vi "Test Publisher.vi"() -> ()   [LabVIEW 2021]
uses:
  ChannelCommon/typedef/FIFO Config.ctl
  ChannelCommon/ChannelCommon.lvlib
  CIFChannels/Typedef/Direction.ctl
  CIFChannels/CIFChannels.lvclass
  CIF_NIChn_Fifo_U8.lvclass
  ChannelCommon/typedef/TimeStamps.ctl
panel:
  in  "stop":bool
  out "timed out?":bool
  out "error out":errorcluster
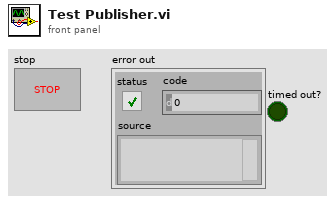
[diagram p1: front panel]
types:
  T1 = typedef "ChannelCommon.lvlib/FIFO Config.ctl" = cluster{"Max Bytes/Msg":u64, "Max Msg/FIFO":u64, "Flags":u64}
  T2 = typedef "CIFChannels.lvclass/Direction.ctl" = enum16{"Publisher", "Subscriber"}
  T3 = typedef "ChannelCommon.lvlib/TimeStamps.ctl" = cluster{"ClockID":u8, "T0":i64, "T_Out":i64}
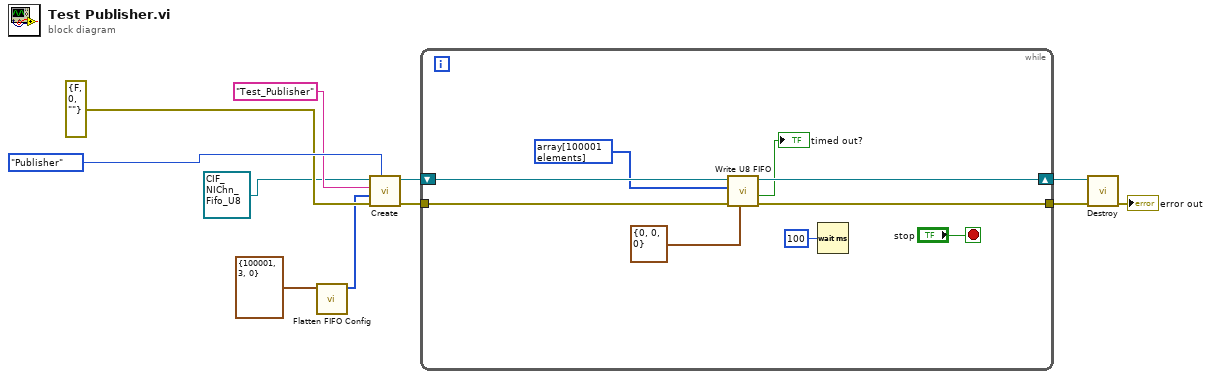
[diagram p0: block diagram]
diagram:
  n1 = call "Flatten FIFO Config.vi"("FIFO Config in"=T1 {"Max Bytes/Msg"=100001, "Max Msg/FIFO"=3, "Flags"=0}) -> ("Flattened FIFO Config"=w1:u8[])  [unwired: 10 in]
  n2 = call-dynamic "Create.vi"("Direction"=Direction."Publisher", "error in (no error)"=errorcluster {"status"=FALSE, "code"=0, "source"=""} ("error out"), "Custom Config Data"=w1, "Name"="Test_Publisher", "CIFFIFO in"=refnum<class "CIF_NIChn_Fifo_U8.lvclass"> refnum ("CIF_NIChn_Fifo_Power.lvclass")) -> ("error out"=w5:errorcluster, "CIFFIFO out"=w6:refnum<class "CIF_NIChn_Fifo_U8.lvclass">)  [unwired: 5 in]
  n3 = while {
    shift-right: [w17] -> w4
    shift-left: w6 -> [w19]
    tunnel: w5 -> [w18]
    tunnel: [w16] -> w3
    stop <- "stop" stop-if-true
    n4 = call "Write U8 FIFO.vi"("FIFO Timestamps"=T3 {"ClockID"=0, "T0"=0, "T_Out"=0}, "error in (no error)"=w18, "U8 Data"=u8[] array[100001 elements], "CIFFIFO in"=w19) -> ("error out"=w16:errorcluster, "timed out?"=→"timed out?":bool, "CIFFIFO out"=w17:refnum<class "CIF_NIChn_Fifo_U8.lvclass">)  [unwired: 5 in]
    n5 = Wait (ms)(milliseconds to wait=u32 100) -> ()  [unwired: 1 out]
  }
  n6 = call-dynamic "Destroy.vi"("error in (no error)"=w3, "CIFFIFO in"=w4) -> ("error out"=→"error out":errorcluster)  [unwired: 8 in, 1 out]
